vi "ifr2025 Parameters.vi"(5 "Logarithmic Increment (2)":dbl=2.0, 6 "Time per Step (50.0)":dbl=50.0, 7 "Step Freq (1.0e3)":dbl=1000.0, 8 "error in (no error)":errorcluster {"code" format="%.0x"}, 9 "Stop Freq (2.4e9)":dbl=2400000000.0, 10 "Start Freq (10.0e3)":dbl=10000.0, 11 "instrument handle":refnum<visa-resource-name>) -> (0 "error out":errorcluster {"code" format="%.0x"}, 3 "instrument handle out":refnum<visa-resource-name>)   [LabVIEW 2009]
doc: "Specify the main sweep parameters."
uses:
  Ifr2025_32.dll
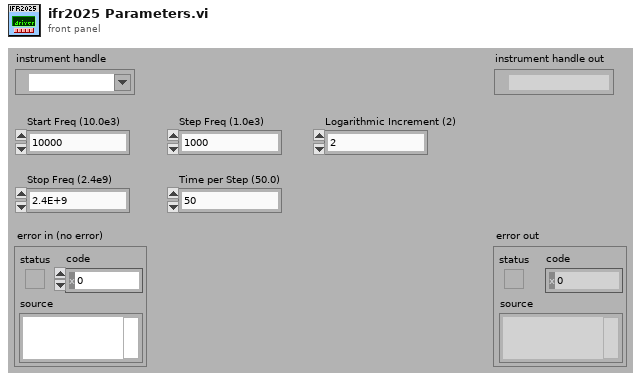
[diagram p1: front panel]
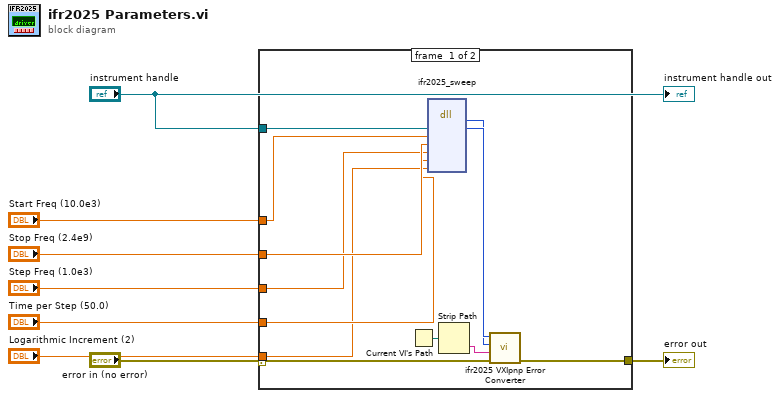
[diagram p0: block diagram]
diagram:
  n1 = case shown="No Error" "error in (no error)" {
    selector: "error in (no error)" -> [w15 w21]
    tunnel: [w14 w21] -> w8
    tunnel: "instrument handle" -> [w19 _]
    tunnel: "Start Freq (10.0e3)" -> [w13 _]
    tunnel: "Stop Freq (2.4e9)" -> [w12 _]
    tunnel: "Step Freq (1.0e3)" -> [w11 _]
    tunnel: "Time per Step (50.0)" -> [w10 _]
    tunnel: "Logarithmic Increment (2)" -> [w9 _]
    frame #0 {
      n2 = Current VI's Path() -> (path=w20:path)
      n3 = dll-call lib="P:/inst/Marconi 2024 Signal Generator/source/labview/ifr2025/ifr2025/ifr2025_*.*" fn="ifr2025_sweep"("vi"=w19, "Start Freq"=w13, "Stop Freq"=w12, "Step Freq"=w11, "Time per Step"=w10, "Logarithmic Increment"=w9) -> (w17:i32, "vi"=w18:u32)  [unwired: 8 in, 2 out]
      n4 = Strip Path(path=w20) -> (name=w16:string)  [unwired: 1 out]
      n5 = call "ifr2025 VXIpnp Error Converter.vi"("error in (no error)"=w15, "name of VI (\"\")"=w16, "CVI error code (0)"=w17, "instrument handle"=w18) -> ("error out"=w14:errorcluster)  [unwired: 7 out]
    }
    frame #1 {
    }
  }
  "error out" <- w8
  "instrument handle out" <- "instrument handle"
